vi "Page_Source_New_Configurable_VI.vi"(8 "error in (no error)":errorcluster, 11 "AB_InteropAssembly in":refnum<class "AB_InteropAssembly.lvclass">) -> (0 "error out":errorcluster, 2 "AB_Source_VI out":refnum<class "AB_Source_VI.lvclass">, 3 "AB_InteropAssembly out":refnum<class "AB_InteropAssembly.lvclass">)   [LabVIEW 2020, in "AB_InteropAssembly.lvclass"]
uses:
  <vilib>/AppBuilder/AB_Classes/InteropAssembly/AB_InteropAssembly.lvclass
  <vilib>/AppBuilder/AB_Classes/Source/VI/AB_Source_VI.lvclass
  <vilib>/AppBuilder/AB_Classes/Source/ExportedAssemblyVI/AB_Source_Exported_Assembly_VI.lvclass
  e:/builds/penguin/labview/branches/2020/dev/dist/vi.lib/AppBuilder/AB_Classes/Source/VI/AB_Source_VI.lvclass
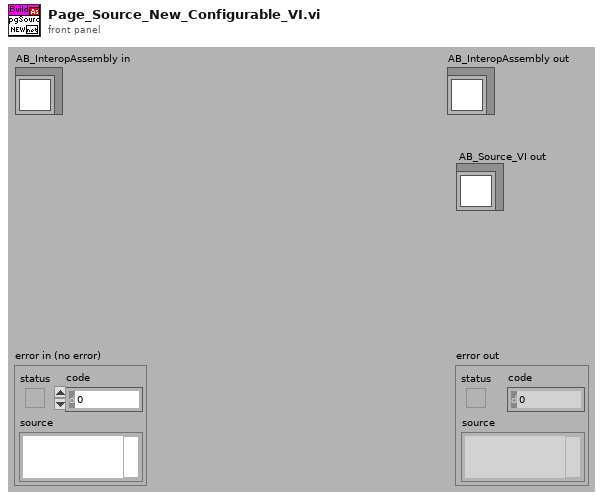
[diagram p1: front panel]
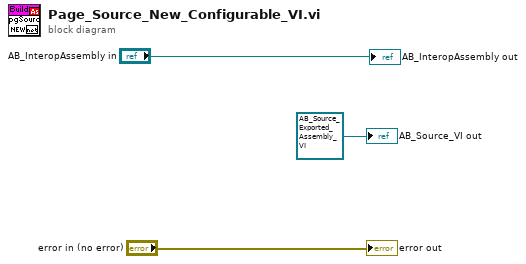
[diagram p0: block diagram]
diagram:
  "error out" <- "error in (no error)"
  "AB_Source_VI out" <- refnum<class "AB_Source_Exported_Assembly_VI.lvclass"> refnum ("AB_Source_Exported_Assembly_VI.lvclass")
  "AB_InteropAssembly out" <- "AB_InteropAssembly in"
